vi "CANOpen_Main_DetectChangevi.vi"(9 "Old":dbl[](array[numeric]), 10 "i":i32, 11 "New":dbl[](array[numeric])) -> (1 "Changed?":bool, 2 "Index":dbl, 3 "Data":dbl)   [LabVIEW 2013, in "CANOpen Addon Custom Device.lvlib"]
uses:
  CANOpen Addon Custom Device.lvlib
  Shared Code/CANOpen_PDO Settings.ctl
  Shared Code/CANOpen_PDO Parameter Settings.ctl
  Shared Code/CANOpen_PDO Data Type.ctl
  System Explorer/SubVIs/CANopen Byte Order.ctl
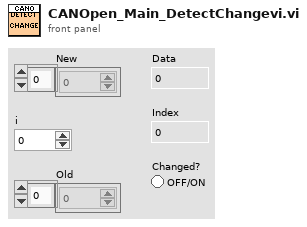
[diagram p1: front panel]
types:
  T1 = typedef "CANOpen Addon Custom Device.lvlib/CANOpen_PDO Settings.ctl" = cluster{"Parameters":T2[], "PDO Channel":u8, "Start Index":u32, "Length":u32}
  T2 = typedef "CANOpen Addon Custom Device.lvlib/CANOpen_PDO Parameter Settings.ctl" = cluster{"Parameter Name":string, "Scale Factor":dbl, "Scale Offset":dbl, "Byte Offset":u8, "Bit Offset":u8, "Data Type":T3, "Byte Order":T4}
  T3 = typedef "CANOpen Addon Custom Device.lvlib/CANOpen_PDO Data Type.ctl" = enum16{"U8", "U16", "U32", "I8", "I16", "I32", "Single", "Double", "Boolean"}
  T4 = typedef "CANOpen Addon Custom Device.lvlib/CANopen Byte Order.ctl" = enum16{"big-endian network order", "little-endian"}
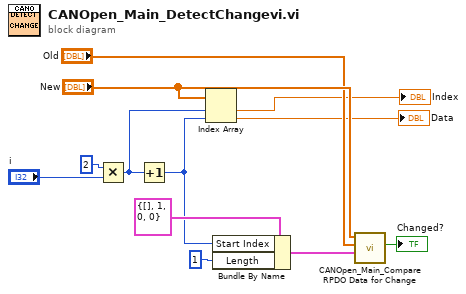
[diagram p0: block diagram]
diagram:
  n1 = Multiply(x=2, y="i") -> (x*y=w9:i32)
  n2 = Increment(x=w9) -> (x+1=w10:i32)
  n3 = Index Array(array="New", index #1=w9, index #2=w10) -> (element #1=→"Index":dbl, element #2=→"Data":dbl)
  n4 = Bundle By Name(cluster=T1 {"Parameters"=[], "PDO Channel"=1, "Start Index"=0, "Length"=0} ("PDO Settings"), "Start Index"=w10, "Length"=u32 1) -> (w5:T1)
  n5 = call "CANOpen_Main_Compare RPDO Data for Change.vi"("PDO Settings"=w5, "Previous Data"="Old", "Current Data"="New") -> ("Changed?"=→"Changed?":bool)  [unwired: 7 in, 1 out]
